vi "Comm_Close.vi"(8 "error in (no error)":errorcluster, 10 "Show Err?":bool=TRUE, 11 "Python in":T1) -> (0 "error out":errorcluster, 2 "return value":string)   [LabVIEW 2022 SP3]
uses:
  PythonCtrl.ctl
  Processors.ctl
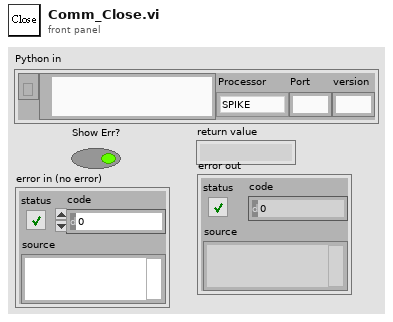
[diagram p1: front panel]
types:
  T1 = typedef "PythonCtrl.ctl" = cluster{"session":refnum<k35>, "PyPath":path, "Processor":T2, "Port":string, "version":string}
  T2 = typedef "Processors.ctl" = enum16{"SPIKE", "Pi", "Pi_ssh", "OpenMV", "Dunio"}
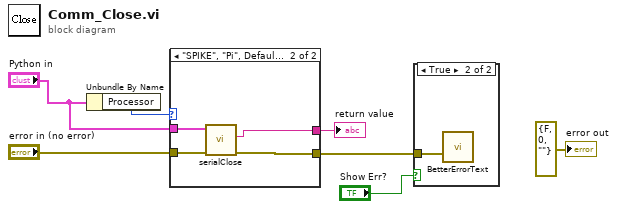
[diagram p0: block diagram]
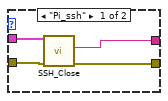
[diagram p3: hidden frame]
diagram:
  n1 = Unbundle By Name("Python in") -> ("Processor"=w5:T2)
  n2 = case shown="\"SPIKE\", \"Pi\", Default" w5 {
    tunnel: "error in (no error)" -> [w11 w15]
    tunnel: [w9 w14] -> w3
    tunnel: "Python in" -> [w10 w13]
    tunnel: [w8 w12] -> w4
    frame "Pi_ssh" {
      n3 = call "SSH_Close.vi"("error in (no error)"=w11, "Python"=w10) -> ("error out"=w9:errorcluster, "return value"=w8:string)  [unwired: 8 in]
    }
    frame "SPIKE", "Pi", Default {
      n4 = call "serialClose.vi"("error in (no error)"=w15, "Python in"=w13) -> ("error out"=w14:errorcluster, "return value"=w12:string)  [unwired: 8 in]
    }
  }
  "return value" <- w4
  n5 = case shown="True" "Show Err?" {
    tunnel: w3 -> [_ w16]
    frame False {
    }
    frame True {
      n6 = call "BetterErrorText.vi"("error in (no error)"=w16) -> ()  [unwired: 9 in, 2 out]
    }
  }
  "error out" <- errorcluster {"status"=FALSE, "code"=0, "source"=""} ("error out")
